vi "defaultdatapathsubvi.vi"(11 "stripped path":path) -> (3 "default data path":path)   [LabVIEW 2018, in "analysis.lvlib"]
uses:
  analysis.lvlib
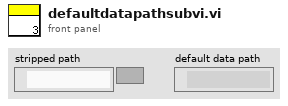
[diagram p1: front panel]
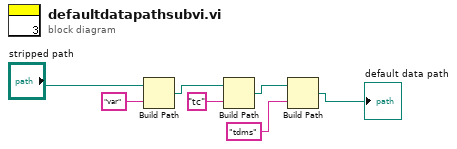
[diagram p0: block diagram]
diagram:
  n1 = Build Path(base path="stripped path", name or relative path="var") -> (appended path=w3:path)
  n2 = Build Path(base path=w3, name or relative path="tc") -> (appended path=w5:path)
  n3 = Build Path(base path=w5, name or relative path="tdms") -> (appended path=→"default data path":path)
